vi "solar_voy_def Export (cmd_tlm).vi"(7 "CMD":enum8{"CMD", "TLM"}(ring), 8 "error in (no error)":errorcluster, 9 "ALL PACKETS":T1[](array[typedef]) {"last_time" format="%<%H:%M:%S%3u %m/%d/%y>T"}, 10 "Target Name":string, 11 "cmd_tlm.txt in":path) -> (0 "error out":errorcluster, 3 "cmd_tlm.txt out":path)   [LabVIEW 2018]
doc: "This exports a Target's packets to the corresponding COSMOS configuration folder:\ncosmos\\config\\targets\\TARGET\\cmd_tlm\\TARGET_cmd|tlm.txt"
uses:
  solar_voy_def_ctl ITEM TYPE.ctl
  type/solar_type Item Type.ctl
  solar_voy_def_ctl ITEM.ctl
  solar_voy_def_ctl PACKET_ID.ctl
  solar_voy_def_ctl PACKET.ctl
panel:
  in  "Suppress Errors? (T)":bool=TRUE
  out "Telemetry":string
  out "Commands":string
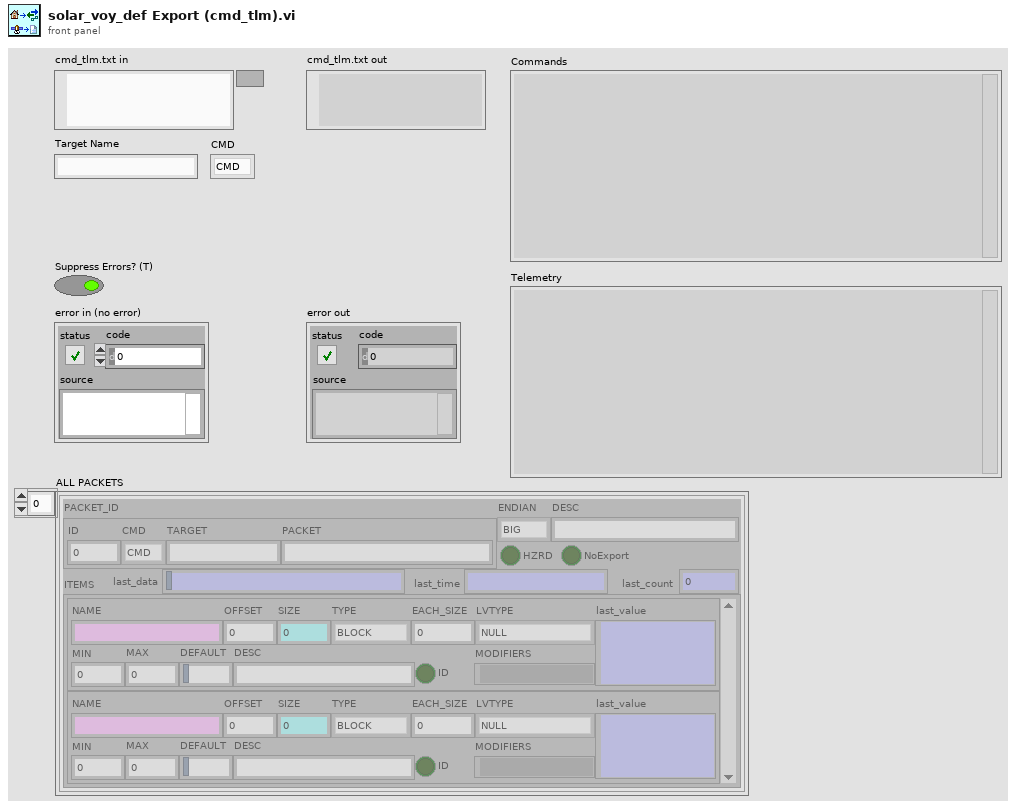
[diagram p1: front panel]
types:
  T1 = typedef "solar_voy_def_ctl PACKET.ctl" = cluster{"PACKET_ID":T2, "ENDIAN":enum8{"BIG", "LITTLE"}, "DESC":string, "HZRD":bool, "ITEMS":T3[], "NoExport":bool, "last_time":timestamp, "last_count":u32, "last_data":string}
  T2 = typedef "solar_voy_def_ctl PACKET_ID.ctl" = cluster{"ID":u16, "CMD":enum8{"CMD", "TLM"}, "TARGET":string, "PACKET":string}
  T3 = typedef "solar_voy_def_ctl ITEM.ctl" = cluster{"NAME":string, "OFFSET":i32, "SIZE":i32, "TYPE":T4, "EACH_SIZE":i32, "LVTYPE":T5, "MIN":dbl, "MAX":dbl, "DEFAULT":string, "DESC":string, "ID":bool, "MODIFIERS":variant, "last_value":variant}
  T4 = typedef "solar_voy_def_ctl ITEM TYPE.ctl" = enum8{"BLOCK", "INT", "UINT", "FLOAT", "STRING"}
  T5 = typedef "solar_type Item Type.ctl" = enum16{"NULL", "UNKNOWN", "CLUSTER", "I8", "I16", "I32", "I64", "U8", "U16", "U32", "U64", "U8_ENUM", "U16_ENUM", "U32_ENUM", "SGL", "DBL", "BOOLEAN", "STRING", "PATH", "VISA", "TAG", "TIME", "I8_1D", "I16_1D", "I32_1D", "I64_1D", "U8_1D", "U16_1D", "U32_1D", "U64_1D", "U8_ENUM_1D", "U16_ENUM_1D", "U32_ENUM_1D", "SGL_1D", "DBL_1D", "BOOLEAN_1D", "STRING_1D", "PATH_1D", "VISA_1D", "TAG_1D", "TIME_1D", "I8_2D", "I16_2D", "I32_2D", "I64_2D", "U8_2D", "U16_2D", "U32_2D", "U64_2D", "U8_ENUM_2D", "U16_ENUM_2D", "U32_ENUM_2D", "SGL_2D", "DBL_2D", "BOOLEAN_2D", "STRING_2D", "PATH_2D", "VISA_2D", "TAG_2D", "TIME_2D"}
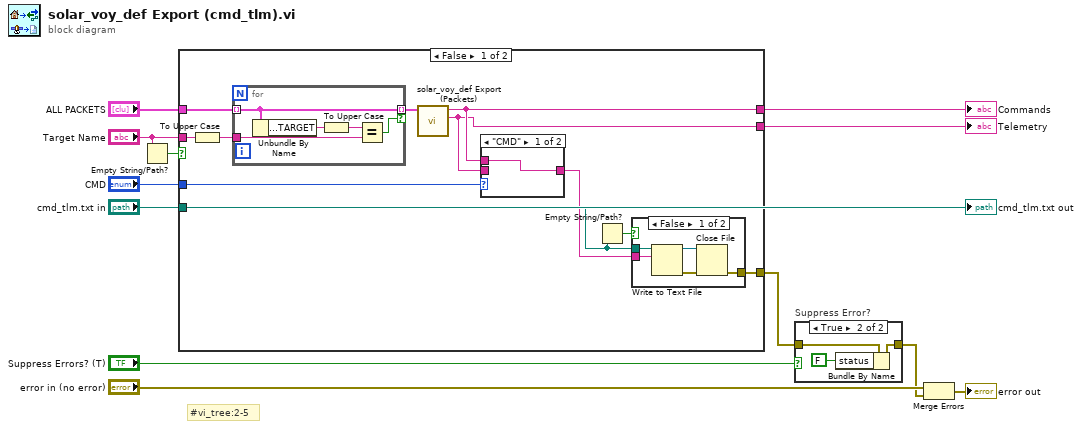
[diagram p0: block diagram]
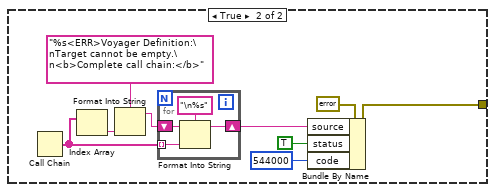
[diagram p4: hidden frame]
diagram:
  # "#vi_tree:2-5"
  n1 = Empty String/Path?(string/path="Target Name") -> (empty?=w1:bool)
  n2 = case shown="False" w1 {
    tunnel: "ALL PACKETS" -> [w23 _]
    tunnel: "Target Name" -> [w21 _]
    tunnel: "CMD" -> [w19 _]
    tunnel: [w18 _] -> w9
    tunnel: [w17 _] -> w8
    tunnel: "cmd_tlm.txt in" -> [w15 _]
    tunnel: [w13 w36] -> w4
    frame False {
      n3 = To Upper Case(1:w21) -> (0:w22:string)
      n4 = for {
        tunnel: w23 -> [w32] mode=indexing
        tunnel: w22 -> [w33]
        tunnel: [w32] -> w20 mode=indexing if=w31
        n5 = Unbundle By Name(w32) -> ("PACKET_ID.TARGET"=w35:string)
        n6 = To Upper Case(1:w35) -> (0:w34:string)
        n7 = Equal?(x=w34, y=w33) -> (x = y?=w31:bool)
      }
      n8 = call "solar_voy_def Export (Packets).vi"("PACKETS"=w20) -> ("Telemetry"=w17:string, "Commands"=w18:string)  [unwired: 9 in]
      n9 = case shown="\"CMD\"" w19 {
        tunnel: w18 -> [w29 _]
        tunnel: w17 -> [_ w30]
        tunnel: [w29 w30] -> w16
        frame "CMD" {
        }
        frame "TLM" {
        }
      }
      n10 = Empty String/Path?(string/path=w15) -> (empty?=w14:bool)
      n11 = case shown="False" w14 {
        tunnel: [w26 _] -> w13
        tunnel: w16 -> [w25 _]
        tunnel: w15 -> [w24 _]
        frame False {
          n12 = Write to Text File(file (use dialog)=w24, text=w25) -> (refnum out=w27:refnum<file>, error out=w28:errorcluster)  [unwired: 2 in, 1 out]
          n13 = Close File(refnum=w27, error in=w28) -> (error out=w26:errorcluster)  [unwired: 1 out]
        }
        frame True {
        }
      }
    }
    frame True {
      n14 = Call Chain() -> (call chain=w39:string[])
      n15 = Index Array(array=w39) -> (element=w41:string)  [unwired: 1 in]
      n16 = Format Into String(format string="%s<ERR>Voyager Definition:\nTarget cannot be empty.\n<b>Complete call chain:</b>", w41) -> (resulting string=w40:string)  [unwired: 2 in, 1 out]
      n17 = for {
        tunnel: w39 -> [w48] mode=indexing
        shift-right: [w47] -> w38
        shift-left: w40 -> [w46]
        n18 = Format Into String(format string="\n%s", initial string=w46, w48) -> (resulting string=w47:string)  [unwired: 1 in, 1 out]
      }
      n19 = Bundle By Name(cluster=errorcluster {"status"=FALSE, "code"=0, "source"=""} ("error in (no error)"), "source"=w38, "status"=TRUE, "code"=544000 ("Code")) -> (w36:errorcluster)
    }
  }
  "Commands" <- w9
  "Telemetry" <- w8
  n20 = case "Suppress Error?" shown="True" "Suppress Errors? (T)" {
    tunnel: w4 -> [w49 w52]
    tunnel: [w49 w51] -> w3
    frame False {
    }
    frame True {
      n21 = Bundle By Name(cluster=w52, "status"=FALSE) -> (w51:errorcluster)
    }
  }
  n22 = Merge Errors("error in (no error)", w3) -> (→"error out":errorcluster)
  "cmd_tlm.txt out" <- "cmd_tlm.txt in"
